vi "Unicode Open File With Filters.vi"() -> ()   [LabVIEW 2020]
uses:
  Types/UTF-8 String/UTF-8 String.lvclass/UTF-8 String.ctl
  Types/UTF-8 Path/UTF-8 Path.lvclass/UTF-8 Path.ctl
  Dialog & User Interface/Polymorphic VIs/Read Control Text/Read String Value (UTF-8 String).vi
  c4007dfa-1da1-44f5-a142-1a1fd44df504.vi
  9673ad0f-ae00-4a53-9a7b-f5b6ad42837e.vi
  Dialog & User Interface/Polymorphic VIs/Write Control Text/Write String Value (UTF-8 String).vi
  Dialog & User Interface/Polymorphic VIs/Read Control Text/Read String Value (UTF-8 String).vi/bfba3187-b22e-4285-8cc2-1816a803f974.vi
  Private/Conversion/String as Encoded String.vi
  Private/Conversion/Polymorphic VIs/String as Encoded String (UTF-8 String).vi
  Private/Conversion/Text as Encoded String.vi
  Private/Conversion/Polymorphic VIs/Text as Encoded String (UTF-8 String).vi
  Private/Library/gu_open_file_dialog.vi
  Private/Library/gu_select_folder_dialog.vi
  Types/UTF-8 Path/Write Encoded UTF-8 Path.vi
  Private/Conversion/Polymorphic VIs/Text as Encoded String (UTF-8 Path).vi
  Types/UTF-8 String/Write Encoded UTF-8 String.vi
  Dialog & User Interface/Polymorphic VIs/Write Control Text/Write String Value (UTF-8 String).vi/5206cb6b-04fb-41f5-a37e-29c14f142303.vi
  Types/UTF-8 String/New UTF-8 String.vi
  Types/UTF-8 String/Read Encoded UTF-8 String.vi
  Private/Memory/Copy String.vi
  Private/Library/Result To Error.vi
  Types/UTF-8 Path/Read Encoded UTF-8 Path.vi
  Private/Conversion/Encoded UTF-8 String to Encoded UTF-16LE String.vi
  Unicode/Encode String.vi
  Private/Memory/Copy String.vi/4d47babd-4a2d-4eb7-b91b-7e707d692665.vi
  Private/Library/gu_free.vi
  Unicode/Detect String Encoding.vi
  Private/Conversion/Text to UTF-8.vi
  Private/Conversion/Polymorphic VIs/Text to UTF-8 (LabVIEW String).vi
  Unicode/SubVIs/UTF-16 Byte Swap.vi
  Private/Conversion/UTF-8 to Text.vi
  Private/Conversion/Polymorphic VIs/UTF-8 to Text (LabVIEW String).vi
  Private/Conversion/Encoded UTF-16LE String to Encoded UTF-8 String.vi
  Unicode/Prepend BOM.vi
  Unicode/Strip BOM.vi
  Unicode/Detect String Encoding.vi/f4e2713d-ca87-487a-b901-d606fc3002c3.vi
  Unicode/SubVIs/Byte Order Marks.vi
  Unicode/Detect BOM.vi
  Private/User Interface/Read String.vi
  Private/Library/gu_is_text_utf16.vi
  Private/Library/gu_is_text_utf8.vi
  <vilib>/Utility/error.llb/Error Cluster From Error Code.vi
  Private/Memory/Copy String Array.vi
  Private/User Interface/Write String.vi
  Types/UTF-8 String/UTF-8 String.lvclass
  Types/UTF-8 Path/UTF-8 Path.lvclass
  G-Unicode.lvlib
panel:
  in  "filter_description":string="*.tif;*.jpg,*.imax;*.png"
  in  "filter_patterns":string="*.tif;*.jpg,*.imax;*.png"
  out "error out":errorcluster
  out "Path out":string
  out "Path":string
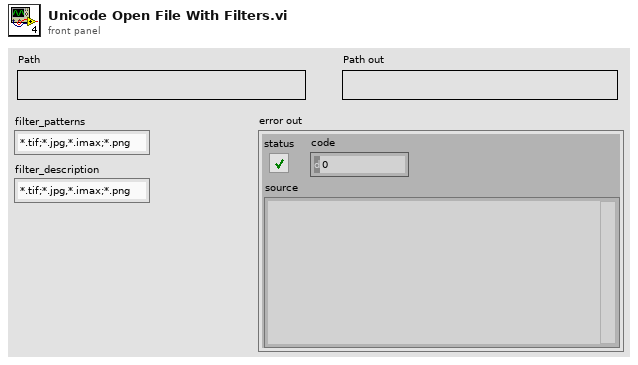
[diagram p1: front panel]
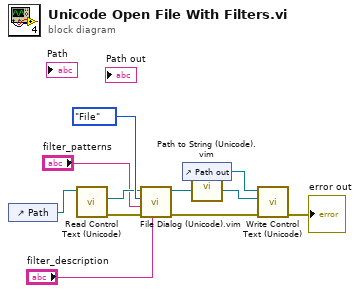
[diagram p0: block diagram]
diagram:
  n1 = control-ref of="Path"() -> (w9:refnum<vi>)
  n2 = call-poly "Read Control Text (Unicode).vi"("Control Ref"=w9) -> ("error out"=w3:errorcluster, "UTF-8 String"=w10:refnum<class "UTF-8 String.lvclass">)  [unwired: 9 in]
  n3 = call "File Dialog (Unicode).vim"("filter_description"="filter_description", "error in"=w3, "filter_patterns"="filter_patterns", "Selection"=enum16{"File", "Multiple Files", "Folder"}."File", "Start Path"=w10) -> ("error out"=w5:errorcluster, "Selected Path"=w7:refnum<class "UTF-8 Path.lvclass">)  [unwired: 3 in, 2 out]
  n4 = control-ref of="Path out"() -> (w8:refnum<vi>)
  n5 = call "Path to String (Unicode).vim"("Path"=w7) -> ("String"=w6:refnum<class "UTF-8 String.lvclass">)  [unwired: 9 in, 1 out]
  n6 = call-poly "Write Control Text (Unicode).vi"("error in"=w5, "Value"=w6, "Control Ref"=w8) -> ("error out"=→"error out":errorcluster)  [unwired: 8 in]
